vi "openMethodViReference.vi"(8 "error in (no error)":errorcluster, 11 "TestCase in":refnum<class "TestCase.lvclass">) -> (0 "error out":errorcluster, 3 "TestCase out":refnum<class "TestCase.lvclass">)   [LabVIEW 2018, in "TestCase.lvclass"]
uses:
  TestCase.lvclass
  TestCase.lvclass/TestCase.ctl
  private/testMethodName.ctl
  JKI Reuse/Filter Error Codes (Scalar)__jki_lib_error_handling -- VI Tester.vi
  Libraries/VITesterUtilities.lvlib
panel:
  # "JKI VI Tester for LabVIEW\nhttp://jkisoft.com/vi-tester\nCopyright (C) 2007-2009, JKI <info@jkisoft.com>\nALL RIGHTS RESERVED"
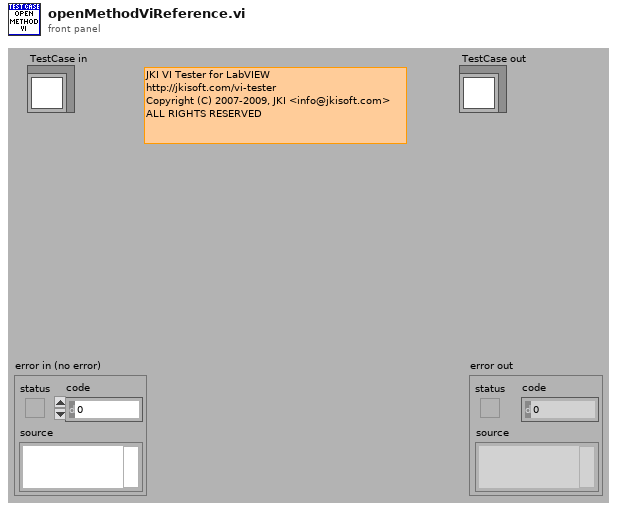
[diagram p1: front panel]
types:
  T1 = typedef "TestCase.lvclass/testMethodName.ctl" = string
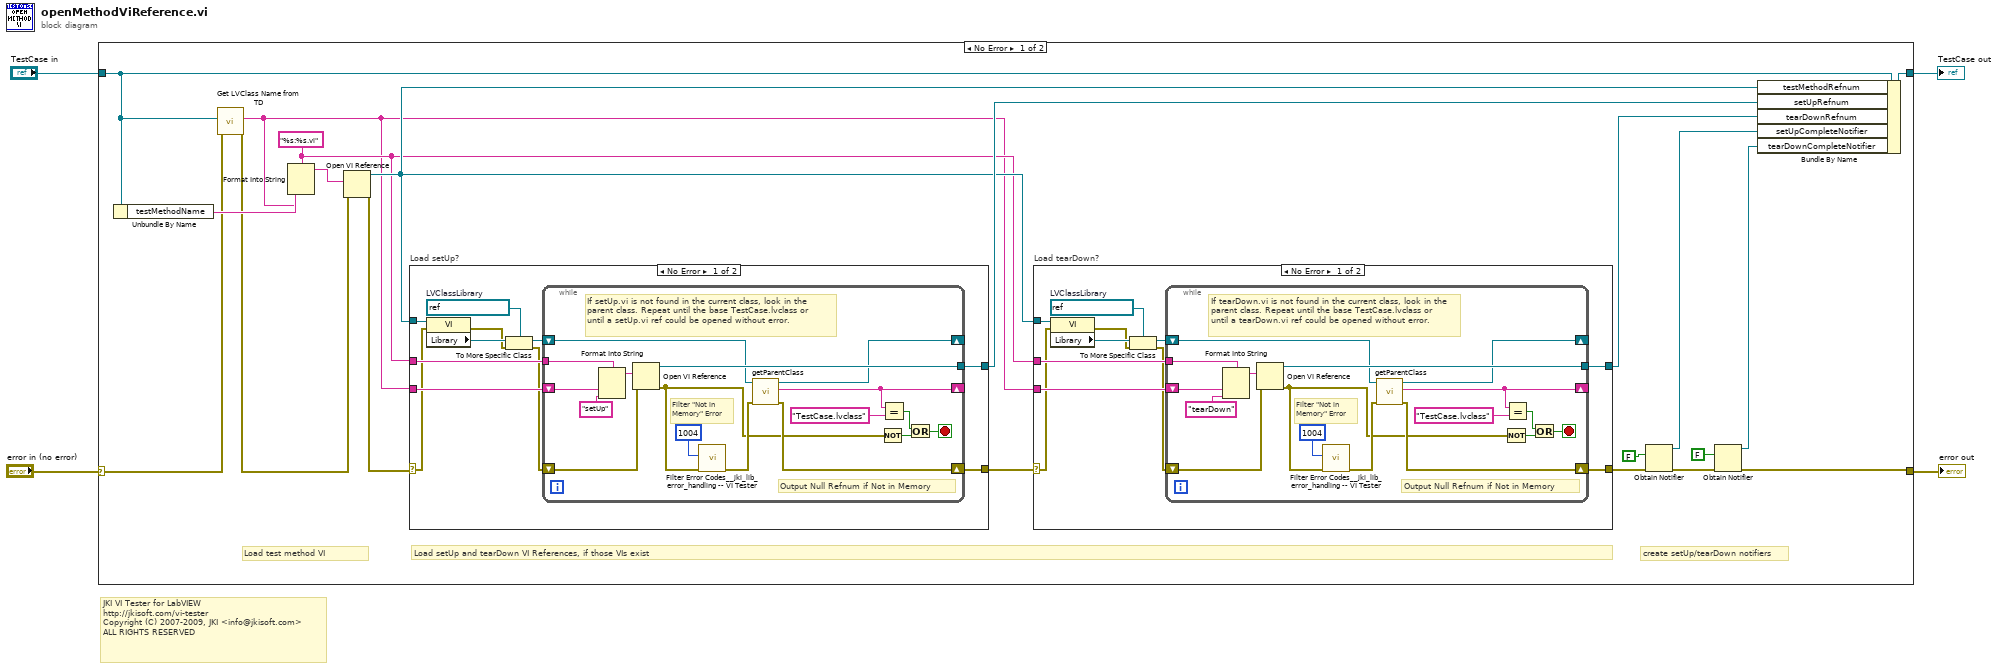
[diagram p0: block diagram]
diagram:
  # "JKI VI Tester for LabVIEW\nhttp://jkisoft.com/vi-tester\nCopyright (C) 2007-2009, JKI <info@jkisoft.com>\nALL RIGHTS RESERVED"
  n1 = case shown="No Error" "error in (no error)" {
    selector: "error in (no error)" -> [w19 w84]
    tunnel: [w13 w84] -> w3
    tunnel: [w21 w83] -> w1
    tunnel: "TestCase in" -> [w20 w83]
    frame No Error {
      w8 = "%s:%s.vi" ("format string")
      # "create setUp/tearDown notifiers"
      # "Load test method VI"
      # "Load setUp and tearDown VI References, if those VIs exist"
      n2 = Unbundle By Name(w20) -> ("testMethodName"=w24:T1)
      n3 = call "Get LVClass Name from TD.vi"("error in"=w19, "Variant"=w20) -> ("error out"=w22:errorcluster, "LVClass Name"=w7:string)  [unwired: 8 in]
      n4 = Format Into String(format string=w8, w7, w24) -> (resulting string=w23:string)  [unwired: 2 in, 1 out]
      n5 = Open VI Reference(vi path=w23, error in (no error)=w22) -> (vi reference=w9:refnum<vi>, error out=w17:errorcluster)  [unwired: 4 in]
      n6 = case "Load setUp?" shown="No Error" w17 {
        selector: w17 -> [w26 w53]
        tunnel: [w35 _] -> w18
        tunnel: w8 -> [w34 _]
        tunnel: [w32 w53] -> w10
        tunnel: w7 -> [w33 _]
        tunnel: w9 -> [w28 _]
        frame No Error {
          w31 = refnum<vi> refnum  # LVClassLibrary
          n7 = property class="VI"(reference=w28, error in=w26) -> (error out=w29:errorcluster, "Library"=w30:refnum<vi>)  [unwired: 1 out]
          n8 = To More Specific Class(target class=w31, reference=w30, error in=w29) -> (specific class reference=w27:refnum<vi>, error out=w25:errorcluster)
          n9 = while {
            tunnel: [w50] -> w35
            tunnel: w34 -> [w49]
            shift-right: [w40] -> w32
            shift-left: w25 -> [w47]
            shift-right: [w44] -> _
            shift-left: w27 -> [w45]
            shift-right: [w43] -> _
            shift-left: w33 -> [w48]
            stop <- w38 stop-if-true
            # "If setUp.vi is not found in the current class, look in the parent class. Repeat until the base TestCase.lvclass or until a setUp.vi ref could be opened without error."
            # "Output Null Refnum if Not in Memory"
            # "Filter \"Not in Memory\" Error"
            n10 = Format Into String(format string=w49, w48, T1 "setUp" ("input 2")) -> (resulting string=w51:string)  [unwired: 2 in, 1 out]
            n11 = Open VI Reference(vi path=w51, error in (no error)=w47) -> (vi reference=w50:refnum<vi>, error out=w37:errorcluster)  [unwired: 4 in]
            n12 = call-poly "Filter Error Codes__jki_lib_error_handling -- VI Tester.vi"("error in"=w37, "error code to filter"=1004) -> ("error out"=w41:errorcluster)  [unwired: 7 in, 2 out]
            n13 = call "getParentClass.vi"("error in (no error)"=w41, "Class Ref"=w45) -> ("error out"=w40:errorcluster, "Parent Class Name"=w43:string, "Parent Class Ref"=w44:refnum<vi>)  [unwired: 7 in]
            n14 = Not(x=w37) -> (.not. x?=w36:bool)
            n15 = Equal?(x=w43, y="TestCase.lvclass") -> (x = y?=w39:bool)
            n16 = Or(x=w39, y=w36) -> (x .or. y?=w38:bool)
          }
        }
        frame Error {
        }
      }
      n17 = case "Load tearDown?" shown="No Error" w10 {
        selector: w10 -> [w55 w82]
        tunnel: [w64 _] -> w5
        tunnel: w8 -> [w63 _]
        tunnel: [w61 w82] -> w6
        tunnel: w7 -> [w62 _]
        tunnel: w9 -> [w57 _]
        frame No Error {
          w60 = refnum<vi> refnum  # LVClassLibrary
          n18 = property class="VI"(reference=w57, error in=w55) -> (error out=w58:errorcluster, "Library"=w59:refnum<vi>)  [unwired: 1 out]
          n19 = To More Specific Class(target class=w60, reference=w59, error in=w58) -> (specific class reference=w56:refnum<vi>, error out=w54:errorcluster)
          n20 = while {
            tunnel: [w79] -> w64
            tunnel: w63 -> [w78]
            shift-right: [w69] -> w61
            shift-left: w54 -> [w76]
            shift-right: [w73] -> _
            shift-left: w56 -> [w74]
            shift-right: [w72] -> _
            shift-left: w62 -> [w77]
            stop <- w67 stop-if-true
            # "If tearDown.vi is not found in the current class, look in the parent class. Repeat until the base TestCase.lvclass or until a tearDown.vi ref could be opened without error."
            # "Output Null Refnum if Not in Memory"
            # "Filter \"Not in Memory\" Error"
            n21 = Format Into String(format string=w78, w77, T1 "tearDown" ("input 2")) -> (resulting string=w80:string)  [unwired: 2 in, 1 out]
            n22 = Open VI Reference(vi path=w80, error in (no error)=w76) -> (vi reference=w79:refnum<vi>, error out=w66:errorcluster)  [unwired: 4 in]
            n23 = call-poly "Filter Error Codes__jki_lib_error_handling -- VI Tester.vi"("error in"=w66, "error code to filter"=1004) -> ("error out"=w70:errorcluster)  [unwired: 7 in, 2 out]
            n24 = call "getParentClass.vi"("error in (no error)"=w70, "Class Ref"=w74) -> ("error out"=w69:errorcluster, "Parent Class Name"=w72:string, "Parent Class Ref"=w73:refnum<vi>)  [unwired: 7 in]
            n25 = Not(x=w66) -> (.not. x?=w65:bool)
            n26 = Equal?(x=w72, y="TestCase.lvclass") -> (x = y?=w68:bool)
            n27 = Or(x=w68, y=w65) -> (x .or. y?=w67:bool)
          }
        }
        frame Error {
        }
      }
      n28 = Obtain Notifier(notification data type=FALSE, error in (no error)=w6) -> (notifier out=w12:refnum<notifier>, error out=w14:errorcluster)  [unwired: 2 in, 1 out]
      n29 = Obtain Notifier(notification data type=FALSE, error in (no error)=w14) -> (notifier out=w11:refnum<notifier>, error out=w13:errorcluster)  [unwired: 2 in, 1 out]
      n30 = Bundle By Name(cluster=w20, "testMethodRefnum"=w9, "setUpRefnum"=w18, "tearDownRefnum"=w5, "setUpCompleteNotifier"=w12, "tearDownCompleteNotifier"=w11) -> (w21:refnum<class "TestCase.lvclass">)
    }
    frame Error {
    }
  }
  "error out" <- w3
  "TestCase out" <- w1
